vi "Take Step.vi"(8 "error in (no error)":errorcluster, 10 "Mouse In":refnum<class "Mouse.lvclass">, 11 "Maze in":refnum<class "Maze.lvclass">) -> (0 "error out":errorcluster, 1 "Bad Action?":bool, 2 "Mouse":refnum<class "Mouse.lvclass">, 3 "Maze":refnum<class "Maze.lvclass">, 4 "New Position":T1, 5 "Direction":T2, 6 "Old Position":T1, 7 "Goal?":bool)   [LabVIEW 2020, in "Maze.lvlib" / "Maze.lvclass"]
doc: "This is the VI meant to be called by the App to progress the exploration by 1 step. It calls into the community scoped Take Step in the mouse class which then manages the mouse state."
uses:
  Maze.lvclass
  Mouse/Mouse.lvclass
  Position.ctl
  Direction.ctl
  Maze.lvclass/Maze.ctl
  Maze.lvlib
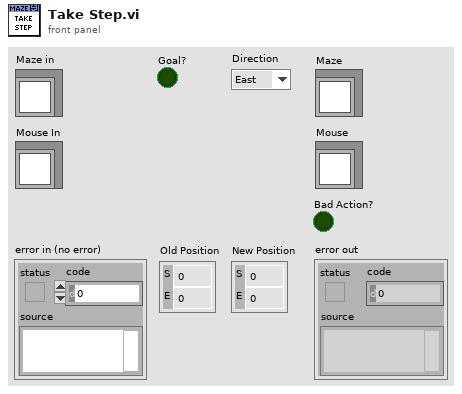
[diagram p1: front panel]
types:
  T1 = typedef "Maze.lvlib/Position.ctl" = cluster{"S":i32, "E":i32}
  T2 = typedef "Maze.lvlib/Direction.ctl" = enum8{"East", "North", "West", "South"}
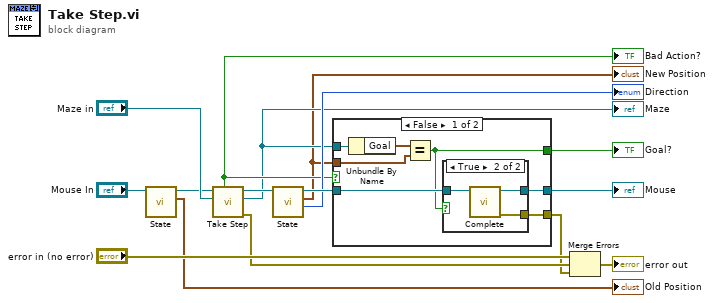
[diagram p0: block diagram]
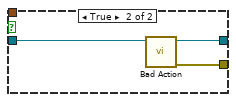
[diagram p3: hidden frame]
diagram:
  n1 = call "State.vi"("Mouse in"="Mouse In") -> ("Position"=→"Old Position":T1, "Mouse out"=w12:refnum<class "Mouse.lvclass">)  [unwired: 7 in, 2 out]
  n2 = call "Take Step.vi"("Maze In"="Maze in", "Mouse in"=w12) -> ("error out"=w6:errorcluster, "Maze"=w4:refnum<class "Maze.lvclass">, "Mouse out"=w8:refnum<class "Mouse.lvclass">, "Bad Action?"=w7:bool)  [unwired: 5 in, 1 out]
  "Bad Action?" <- w7
  "Maze" <- w4
  n3 = call "State.vi"("Mouse in"=w8) -> ("Direction"=→"Direction":T2, "Position"=w3:T1, "Mouse out"=w10:refnum<class "Mouse.lvclass">)  [unwired: 7 in, 1 out]
  "New Position" <- w3
  n4 = case shown="False" w7 {
    tunnel: w10 -> [w20 w30]
    tunnel: [w18 w29] -> w1
    tunnel: [w19 w28] -> w5
    tunnel: w4 -> [w23 _]
    tunnel: w3 -> [w21 _]
    tunnel: [w17 _] -> w2
    frame False {
      n5 = Unbundle By Name(w23) -> ("Goal"=w22:T1)
      n6 = Equal?(x=w22, y=w21) -> (x = y?=w17:bool)
      n7 = case shown="True" w17 {
        tunnel: w20 -> [w24 w27]
        tunnel: [w24 w26] -> w19
        tunnel: [_ w25] -> w18
        frame False {
        }
        frame True {
          n8 = call-dynamic "Complete.vi"("Mouse in"=w27) -> ("error out"=w25:errorcluster, "Mouse out"=w26:refnum<class "Mouse.lvclass">)  [unwired: 9 in]
        }
      }
    }
    frame True {
      n9 = call-dynamic "Bad Action.vi"("Mouse in"=w30) -> ("error out"=w29:errorcluster, "Mouse out"=w28:refnum<class "Mouse.lvclass">)  [unwired: 9 in]
    }
  }
  "Mouse" <- w5
  "Goal?" <- w2
  n10 = Merge Errors("error in (no error)", w6, w1) -> (→"error out":errorcluster)
